vi "ENG_Acquire CI and AI.vi"   [LabVIEW 2017]
uses:
  widgets/EnumStateMachine.llb/AcquireData_Enum.ctl
  widgets/EnumStateMachine.llb/RunTest_Enum.ctl
  <vilib>/DAQmx/read.llb/DAQmx Read (Counter DBL 1Chan 1Samp).vi
  <vilib>/DAQmx/read.llb/DAQmx Read (Analog 2D DBL NChan NSamp).vi
  <vilib>/Analysis/baseanly.llb/Mean (DBL).vi
  widgets/EnumStateMachine.llb/AcquireData_InsertQueues.vi
  widgets/EnumStateMachine.llb/AcquireData_RemoveQueue.vi
  <vilib>/DAQmx/miscellaneous.llb/DAQmx Fill In Error Info.vi
  widgets/EnumStateMachine.llb/RunTest_InsertQueues.vi
  Share data/Default volues.vi
  <vilib>/DAQmx/create/channels.llb/DAQmx Create Channel (CI-Position-Linear Encoder).vi
  <vilib>/DAQmx/configure/timing.llb/DAQmx Timing (Sample Clock).vi
  <vilib>/DAQmx/create/channels.llb/DAQmx Create Channel (AI-Voltage-Basic).vi
  <vilib>/Analysis/NI_AALBase.lvlib
  <resource>/objmgr/daqmx.rc
types:
  T1 = typedef "AcquireData_Enum.ctl" = enum16{"Core: Idle", "Core: Initialize", "Core: Error handle", "Core: Data prepare", "StartAcquire", "StopAcquire", "Core: Exit"}
  T2 = typedef "Queue RefNum" = refnum<k1>
  T3 = typedef "RunTest_Enum.ctl" = enum16{"Core: Idle", "Core: Initialize", "Core: Error handle", "Core: Data prepare", "Core: Exit", "Event: Running ", "Event: Direction", "Event: Danger", "Event: SaveMode", "Event: ManualSave", "Comm: Acquiring"}
  T4 = cluster{"AI Channel":tag, "Min Voltage":dbl, "Max Voltage":dbl, "Terminal Configuration":i32, "Sample Rate":dbl, "Number of Samples":i32, "Logging Mode":i32, "TDMS File Path":path, "Digital Start Trigger Source":tag, "Digital Start Trigger Edge":i32}
  T5 = cluster{"Counter":tag, "A Input Terminal":tag, "B Input Terminal":tag, "Z Index Enable":bool, "Z Index Terminal":tag, "Sample Clock Source":tag, "Sample Rate":dbl, "Samples per Loop":i32, "Digital Trigger Source":tag, "Edge":i32, "distance per pulse":dbl, "initial position":dbl}
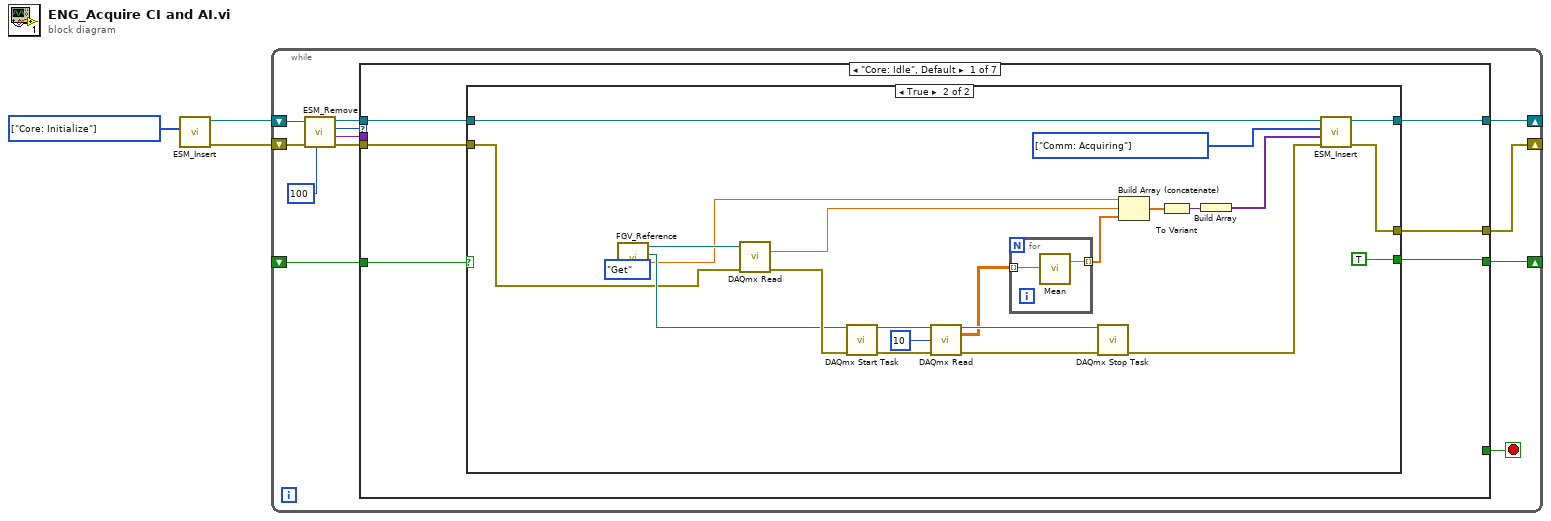
[diagram p0: block diagram]
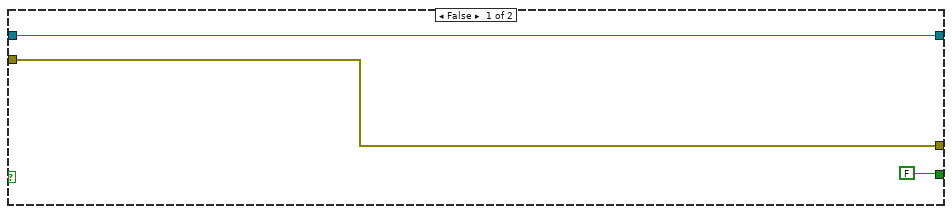
[diagram p2: hidden frame]
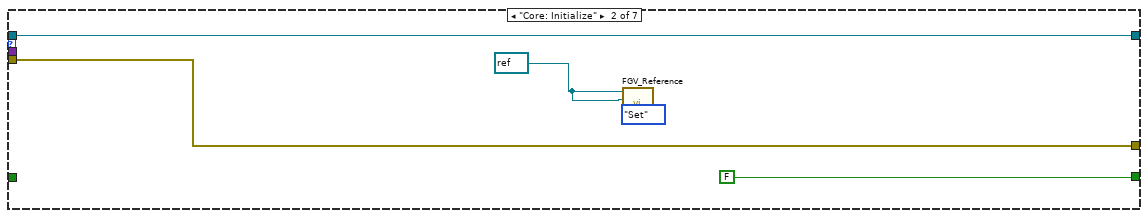
[diagram p3: hidden frame]
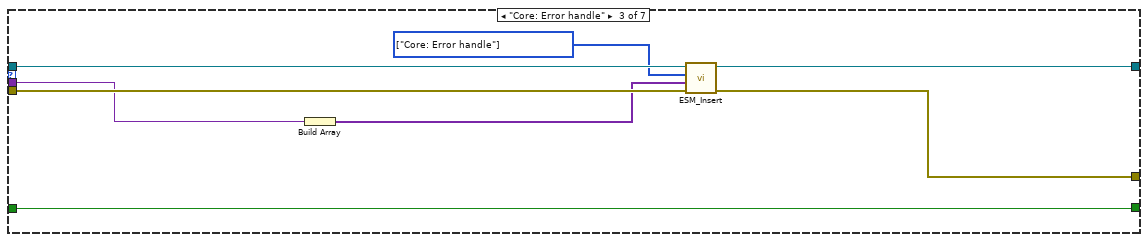
[diagram p4: hidden frame]
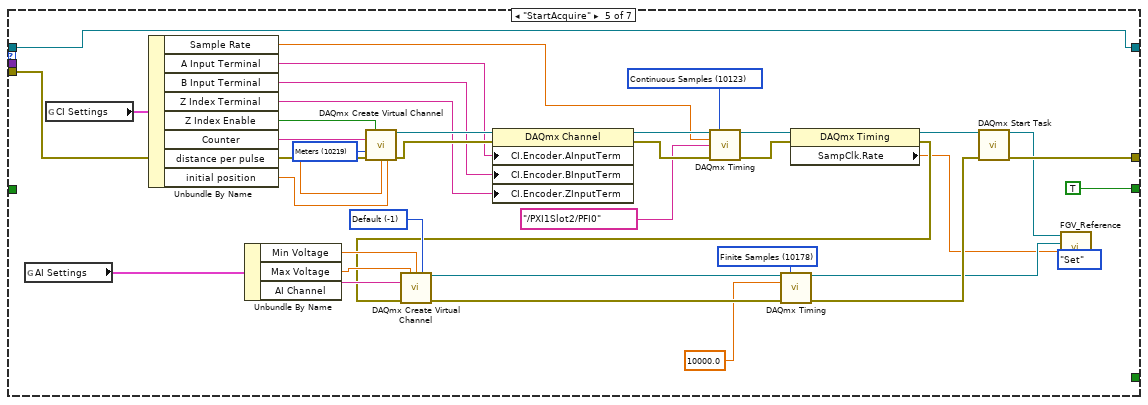
[diagram p6: hidden frame]
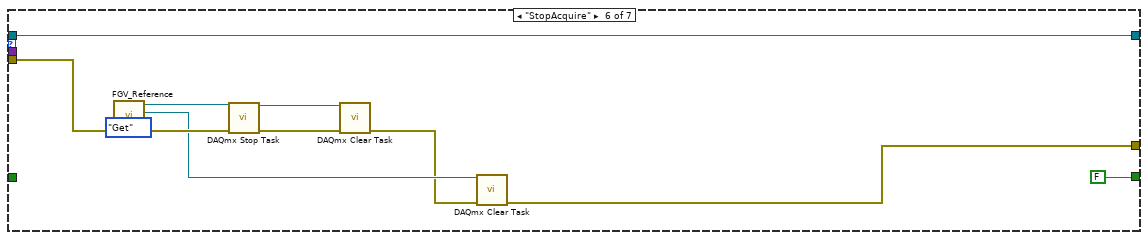
[diagram p7: hidden frame]
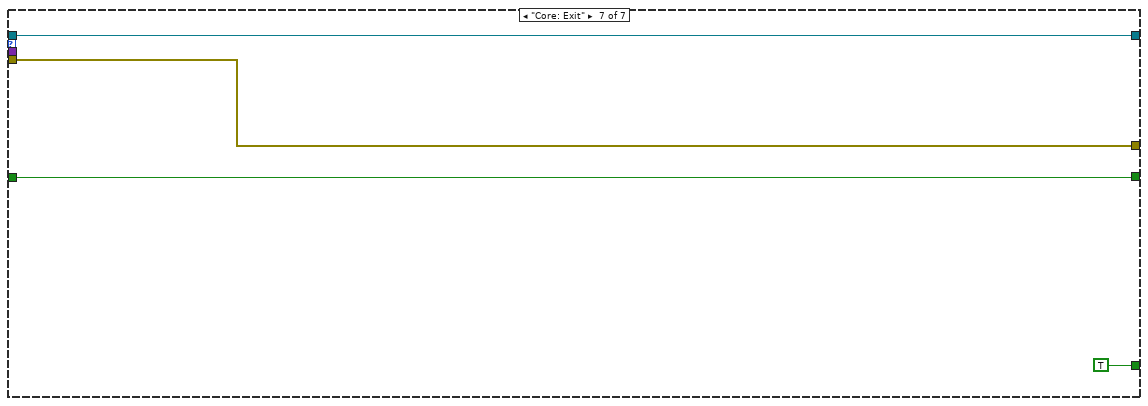
[diagram p8: hidden frame]
diagram:
  w3 = T1[] [enum."Core: Initialize"] items=["Core: Idle", "Core: Initialize", "Core: Error handle", "Core: Data prepare", "StartAcquire", "StopAcquire", "Core: Exit"] ("Templates")
  n1 = call-poly "ESM_Insert.vi"("Templates"=w3) -> ("error out"=w1:errorcluster, "queue out"=w2:T2)  [unwired: 9 in]
  n2 = while {
    shift-right: [w5] -> _
    shift-left: w2 -> [w14]
    shift-right: [w8] -> _
    shift-left: w1 -> [w15]
    shift-right: [w7] -> _
    shift-left: _ -> [w6]
    stop <- w4 stop-if-true
    n3 = call-poly "ESM_Remove.vi"("ms timeout (-1)"=100, "error in (no error)"=w15, "queue"=w14) -> ("错误输出"=w10:errorcluster, "data"=w11:variant, "Template out"=w12:T1, "queue out"=w9:T2)  [unwired: 5 in]
    n4 = case shown="\"Core: Idle\", Default" w12 {
      tunnel: w11 -> [_ _ w57 _ _ _ _]
      tunnel: w10 -> [w19 w52 w60 w63 w103 w109 w116]
      tunnel: w9 -> [w20 w53 w61 w65 w73 w113 w117]
      tunnel: [w18 w52 w59 w63 w95 w104 w116] -> w8
      tunnel: [w17 FALSE w62 w64 TRUE FALSE w115] -> w7
      tunnel: w6 -> [w21 _ w62 w64 _ _ w115]
      tunnel: [w16 w53 w58 w65 w73 w113 w117] -> w5
      tunnel: [_ _ _ _ _ _ TRUE] -> w4
      frame "Core: Idle", Default {
        n5 = case shown="True" w21 {
          tunnel: w20 -> [w22 w37]
          tunnel: w19 -> [w23 w28]
          tunnel: [w23 w34] -> w18
          tunnel: [FALSE TRUE] -> w17
          tunnel: [w22 w36] -> w16
          frame False {
          }
          frame True {
            w33 = T3[] [enum."Comm: Acquiring"] items=["Core: Idle", "Core: Initialize", "Core: Error handle", "Core: Data prepare", "Core: Exit", "Event: Running ", "Event: Direction", "Event: Danger", "Event: SaveMode", "Event: ManualSave", "Comm: Acquiring"] ("SV_RunTest")
            n6 = call "FGV_Reference.vi"("FV_Acquire"=enum16{"Set", "Get"}."Get") -> ("Real Rate Out"=w31:dbl, "CoilVolte Out"=w44:refnum<k21>, "LineEncoder Out"=w46:refnum<k21>)  [unwired: 8 in]
            n7 = call-poly <vilib>:"DAQmx Read.vi"("task/channels in"=w46, "error in"=w28) -> ("data"=w30:dbl, "error out"=w45:errorcluster)  [unwired: 11 in, 1 out]
            n8 = call <vilib>:"DAQmx Start Task.vi"("task/channels in"=w44, "error in"=w45) -> ("task out"=w43:refnum<k21>, "error out"=w42:errorcluster)  [unwired: 12 in]
            n9 = call-poly <vilib>:"DAQmx Read.vi"("task/channels in"=w43, "number of samples per channel"=10, "error in"=w42) -> ("task out"=w40:refnum<k21>, "data"=w32:dbl[][], "error out"=w39:errorcluster)  [unwired: 10 in]
            n10 = for {
              tunnel: w32 -> [w49] mode=indexing
              tunnel: [w48] -> w29 mode=indexing
              n11 = call-poly <vilib>:"Mean.vi"("X"=w49) -> ("mean"=w48:dbl)  [unwired: 1 out]
            }
            n12 = call <vilib>:"DAQmx Stop Task.vi"("task/channels in"=w40, "error in"=w39) -> ("error out"=w35:errorcluster)  [unwired: 12 in, 1 out]
            n13 = Build Array (concatenate)(w31, w30, w29) -> (w27:dbl[])
            n14 = To Variant(anything=w27) -> (Variant=w26:variant)
            n15 = Build Array(w26) -> (w25:variant[])
            n16 = call-poly "ESM_Insert.vi"("error in (no error)"=w35, "datas"=w25, "SV_RunTest"=w33, "queue"=w37) -> ("error out"=w34:errorcluster, "queue out"=w36:T2)  [unwired: 6 in]
          }
        }
      }
      frame "Core: Initialize" {
        w50 = refnum<k21> refnum ("LineEncoder  In")
        n17 = call "FGV_Reference.vi"("FV_Acquire"=enum16{"Set", "Get"}."Set", "CoilVolte In"=w50, "LineEncoder  In"=w50) -> ()  [unwired: 6 in, 3 out]
      }
      frame "Core: Error handle" {
        w55 = T3[] [enum."Core: Error handle"] items=["Core: Idle", "Core: Initialize", "Core: Error handle", "Core: Data prepare", "Core: Exit", "Event: Running ", "Event: Direction", "Event: Danger", "Event: SaveMode", "Event: ManualSave", "Comm: Acquiring"] ("SV_RunTest")
        n18 = Build Array(w57) -> (w56:variant[])
        n19 = call-poly "ESM_Insert.vi"("error in (no error)"=w60, "datas"=w56, "SV_RunTest"=w55, "queue"=w61) -> ("error out"=w59:errorcluster, "queue out"=w58:T2)  [unwired: 6 in]
      }
      frame "Core: Data prepare" {
      }
      frame "StartAcquire" {
        w78 = 10219 items=["Meters"=10219, "Inches"=10379, "Ticks"=10304, "From Custom Scale"=10065] ("units")
        w85 = -1 items=["Default"=-1, "RSE"=10083, "NRSE"=10078, "Differential"=10106, "Pseudodifferential"=12529] ("input terminal configuration")
        w98 = 10178 items=["Finite Samples"=10178, "Continuous Samples"=10123, "Hardware Timed Single Point"=12522] ("sample mode")
        w102 = 10123 items=["Finite Samples"=10178, "Continuous Samples"=10123, "Hardware Timed Single Point"=12522] ("sample mode")
        n20 = global read "Default volues.vi" "AI Settings"() -> (w89:T4)
        n21 = global read "Default volues.vi" "CI Settings"() -> (w84:T5)
        n22 = Unbundle By Name(w84) -> ("Sample Rate"=w71:dbl, "A Input Terminal"=w81:tag, "B Input Terminal"=w82:tag, "Z Index Terminal"=w83:tag, "Z Index Enable"=w80:bool, "Counter"=w79:tag, "distance per pulse"=w75:dbl, "initial position"=w74:dbl)
        n23 = Unbundle By Name(w89) -> ("Min Voltage"=w87:dbl, "Max Voltage"=w86:dbl, "AI Channel"=w88:tag)
        n24 = call-poly <vilib>:"DAQmx Create Virtual Channel.vi"("z index enable"=w80, "counter"=w79, "units"=w78, "error in"=w103, "distance per pulse"=w75, "initial position"=w74) -> ("task out"=w101:refnum<k21>, "error out"=w91:errorcluster)  [unwired: 8 in]
        n25 = property class="DAQmx Channel"(reference=w101, error in=w91, "CI.Encoder.AInputTerm"=w81, "CI.Encoder.BInputTerm"=w82, "CI.Encoder.ZInputTerm"=w83) -> (reference out=w92:refnum<k21>, error out=w90:errorcluster)
        n26 = call-poly <vilib>:"DAQmx Timing.vi"("task/channels in"=w92, "sample mode"=w102, "rate"=w71, "source"=tag "/PXI1Slot2/PFI0", "error in"=w90) -> ("task out"=w72:refnum<k21>, "error out"=w69:errorcluster)  [unwired: 9 in]
        n27 = property class="DAQmx Timing"(reference=w72, error in=w69) -> (reference out=w70:refnum<k21>, error out=w68:errorcluster, "SampClk.Rate"=w67:dbl)
        n28 = call-poly <vilib>:"DAQmx Create Virtual Channel.vi"("maximum value"=w86, "minimum value"=w87, "input terminal configuration"=w85, "physical channels"=w88, "error in"=w68) -> ("task out"=w100:refnum<k21>, "error out"=w99:errorcluster)  [unwired: 9 in]
        n29 = call-poly <vilib>:"DAQmx Timing.vi"("task/channels in"=w100, "sample mode"=w98, "rate"=10000.0, "error in"=w99) -> ("task out"=w76:refnum<k21>, "error out"=w96:errorcluster)  [unwired: 10 in]
        n30 = call <vilib>:"DAQmx Start Task.vi"("task/channels in"=w70, "error in"=w96) -> ("task out"=w77:refnum<k21>, "error out"=w95:errorcluster)  [unwired: 12 in]
        n31 = call "FGV_Reference.vi"("FV_Acquire"=enum16{"Set", "Get"}."Set", "Real Rate In"=w67, "CoilVolte In"=w76, "LineEncoder  In"=w77) -> ()  [unwired: 5 in, 3 out]
      }
      frame "StopAcquire" {
        n32 = call "FGV_Reference.vi"("FV_Acquire"=enum16{"Set", "Get"}."Get") -> ("CoilVolte Out"=w106:refnum<k21>, "LineEncoder Out"=w110:refnum<k21>)  [unwired: 8 in, 1 out]
        n33 = call <vilib>:"DAQmx Stop Task.vi"("task/channels in"=w110, "error in"=w109) -> ("task out"=w108:refnum<k21>, "error out"=w107:errorcluster)  [unwired: 12 in]
        n34 = call <vilib>:"DAQmx Clear Task.vi"("task in"=w108, "error in"=w107) -> ("error out"=w105:errorcluster)  [unwired: 13 in]
        n35 = call <vilib>:"DAQmx Clear Task.vi"("task in"=w106, "error in"=w105) -> ("error out"=w104:errorcluster)  [unwired: 13 in]
      }
      frame "Core: Exit" {
      }
    }
  }
